vi "Get UART Channel Name.vi"(7 "UART Channel Names":string[](array[string]), 8 "Error In":errorcluster, 10 "UART Channel":u8) -> (0 "Error Out":errorcluster, 2 "UART Channel":string)   [LabVIEW 2013, in "LVH-LINX.lvlib" / "myRIO.lvlib"]
uses:
  <vilib>/LabVIEW Hacker/LINX/Private/myRIO/myRIO.lvlib
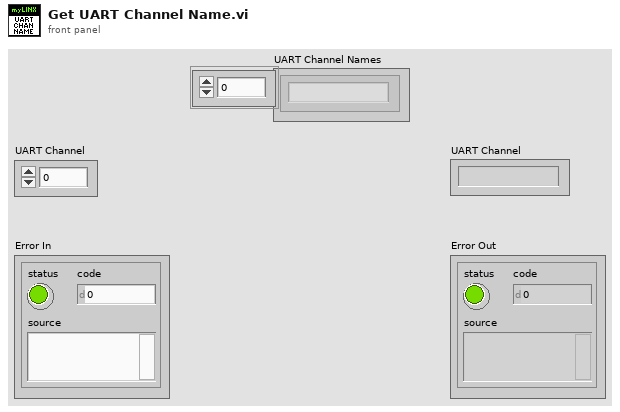
[diagram p1: front panel]
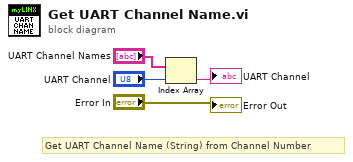
[diagram p0: block diagram]
diagram:
  # "Get UART Channel Name (String) from Channel Number"
  n1 = Index Array(array="UART Channel Names", index="UART Channel") -> (element=→"UART Channel":string)
  "Error Out" <- "Error In"
